vi "LM_fit.vi"(8 "Error In":errorcluster, 10 "Intensities":dbl[](array[numeric]), 11 "Angles":dbl[](array[numeric])) -> (0 "Error Out":errorcluster, 1 "Extinction Angle":dbl, 2 "best fit parameters":dbl[](array[numeric]), 3 "best nonlinear fit":dbl[](array[numeric]))   [LabVIEW 2019]
uses:
  <vilib>/gmath/NumericalOptimization/Nonlinear Curve Fit LM.vi
  <vilib>/gmath/NI_Gmath.lvlib
panel:
  out "XY Graph":cluster{"Angles":dbl[], "Intensities":dbl[]}[](graph)
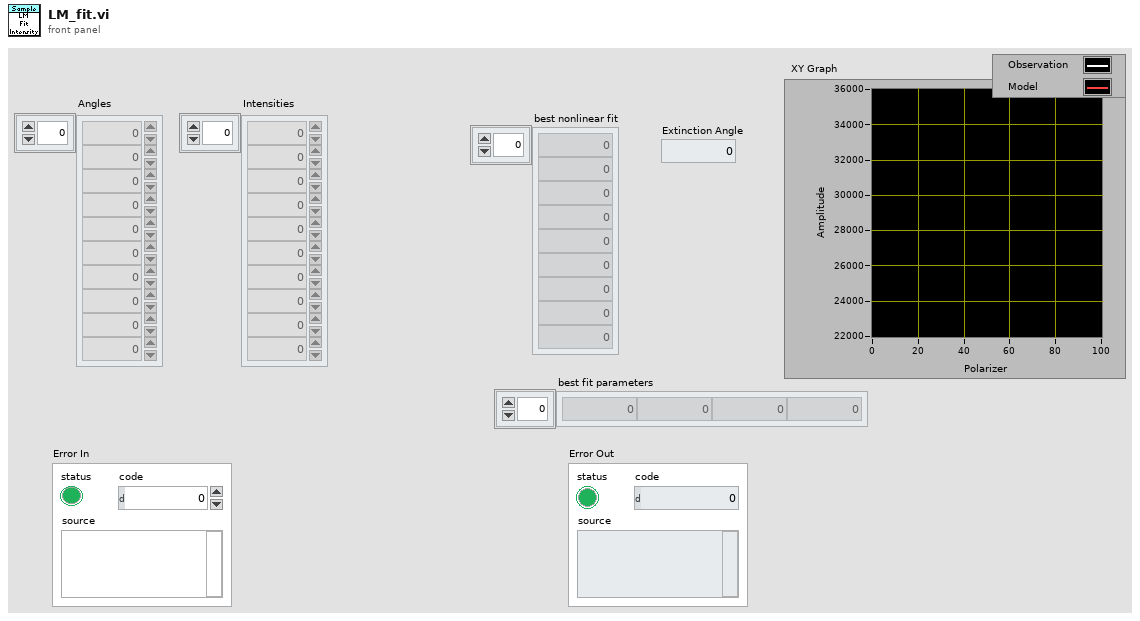
[diagram p1: front panel]
types:
  T1 = cluster{"Angles":dbl[], "best nonlinear fit":dbl[]}
  T2 = cluster{"Angles":dbl[], "best nonlinear fit":dbl[]}[]
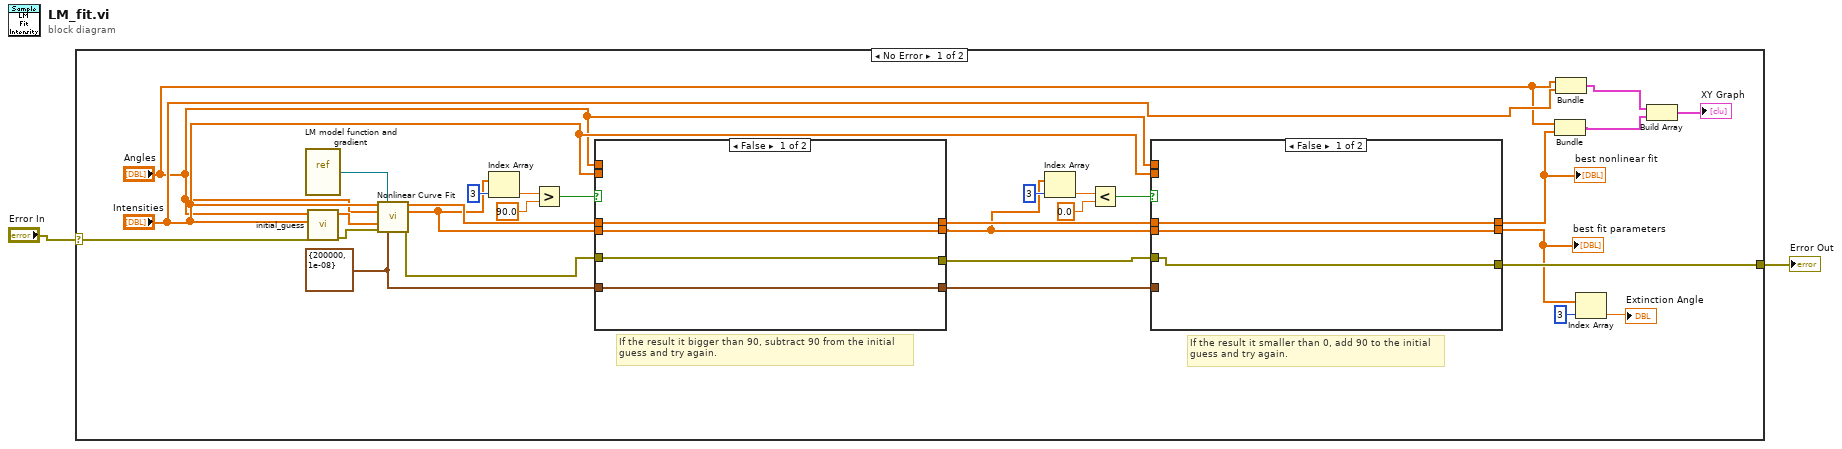
[diagram p0: block diagram]
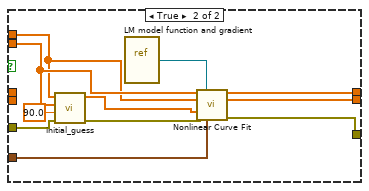
[diagram p2: hidden frame]
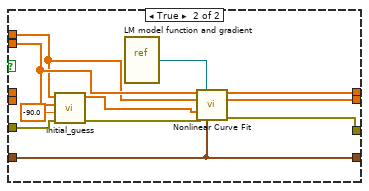
[diagram p3: hidden frame]
diagram:
  n1 = case shown="No Error" "Error In" {
    selector: "Error In" -> [w15 w62]
    tunnel: [w14 w62] -> w1
    frame No Error {
      w10 = cluster{"max iteration":i32, "tolerance":dbl} {"max iteration"=200000, "tolerance"=1e-08} ("termination")
      # "If the result it smaller than 0, add 90 to the initial\nguess and try again."
      # "If the result it bigger than 90, subtract 90 from the initial\nguess and try again."
      n2 = vi-ref "LM model function and gradient.vi"() -> (w32:refnum<vi>)
      n3 = call "initial_guess.vi"("Error In"=w15, "Intensities"="Intensities", "Angles"="Angles") -> ("Error Out"=w26:errorcluster, "Guess"=w31:dbl[])  [unwired: 7 in]
      n4 = call-poly <vilib>:"Nonlinear Curve Fit.vi"("Y"="Intensities", "f(x,a)"=w32, "X"="Angles", "initial parameters"=w31, "error in (no error)"=w26, "termination"=w10) -> ("best nonlinear fit"=w24:dbl[], "best fit parameters"=w23:dbl[], "error out"=w25:errorcluster)  [unwired: 4 in, 3 out]
      n5 = Index Array(array=w23, index=3) -> (element=w29:dbl)
      n6 = Greater?(x=w29, y=90.0) -> (0:w27:bool)
      n7 = case shown="False" w27 {
        tunnel: "Angles" -> [_ w57]
        tunnel: "Intensities" -> [_ w58]
        tunnel: w25 -> [w48 w59]
        tunnel: [w50 w54] -> w18
        tunnel: [w49 w53] -> w16
        tunnel: w24 -> [w50 _]
        tunnel: w23 -> [w49 _]
        tunnel: [w48 w52] -> w17
        tunnel: w10 -> [w47 w51]
        tunnel: [w47 w51] -> w9
        frame False {
        }
        frame True {
          n8 = call "initial_guess.vi"("Error In"=w59, "Angle Guess Offset"=-90.0, "Intensities"=w58, "Angles"=w57) -> ("Error Out"=w55:errorcluster, "Guess"=w56:dbl[])  [unwired: 6 in]
          n9 = vi-ref "LM model function and gradient.vi"() -> (w61:refnum<vi>)
          n10 = call-poly <vilib>:"Nonlinear Curve Fit.vi"("Y"=w58, "f(x,a)"=w61, "X"=w57, "initial parameters"=w56, "error in (no error)"=w55, "termination"=w51) -> ("best nonlinear fit"=w54:dbl[], "best fit parameters"=w53:dbl[], "error out"=w52:errorcluster)  [unwired: 4 in, 3 out]
        }
      }
      n11 = Index Array(array=w16, index=3) -> (element=w20:dbl)
      n12 = Less?(x=w20, y=0.0) -> (x < y?=w22:bool)
      n13 = case shown="False" w22 {
        tunnel: "Angles" -> [_ w42]
        tunnel: "Intensities" -> [_ w43]
        tunnel: w17 -> [w33 w44]
        tunnel: [w35 w39] -> w4
        tunnel: [w34 w38] -> w13
        tunnel: w18 -> [w35 _]
        tunnel: w16 -> [w34 _]
        tunnel: [w33 w37] -> w14
        tunnel: w9 -> [_ w36]
        frame False {
        }
        frame True {
          n14 = call "initial_guess.vi"("Error In"=w44, "Angle Guess Offset"=90.0, "Intensities"=w43, "Angles"=w42) -> ("Error Out"=w40:errorcluster, "Guess"=w41:dbl[])  [unwired: 6 in]
          n15 = vi-ref "LM model function and gradient.vi"() -> (w46:refnum<vi>)
          n16 = call-poly <vilib>:"Nonlinear Curve Fit.vi"("Y"=w43, "f(x,a)"=w46, "X"=w42, "initial parameters"=w41, "error in (no error)"=w40, "termination"=w36) -> ("best nonlinear fit"=w39:dbl[], "best fit parameters"=w38:dbl[], "error out"=w37:errorcluster)  [unwired: 4 in, 3 out]
        }
      }
      "best nonlinear fit" <- w4
      "best fit parameters" <- w13
      n17 = Bundle("Angles"="Angles", "best nonlinear fit"=w4) -> (w3:T1)  [unwired: 1 in]
      n18 = Bundle("Angles"="Angles", "Intensities"="Intensities") -> (w7:cluster{"Angles":dbl[], "Intensities":dbl[]})  [unwired: 1 in]
      n19 = Index Array(array=w13, index=3) -> (element=→"Extinction Angle":dbl)
      n20 = Build Array(w7, w3) -> (→"XY Graph":T2)
    }
    frame Error {
    }
  }
  "Error Out" <- w1
